vi "Open FP.vi"(8 "error in (no error)":errorcluster, 11 "AMS Gas Actor in":refnum<class "AMS Gas Actor.lvclass">=refnum) -> (0 "error out":errorcluster, 3 "AMS Gas Actor out":refnum<class "AMS Gas Actor.lvclass">)   [LabVIEW 2015]
uses:
  AMS Gas Actor.lvclass
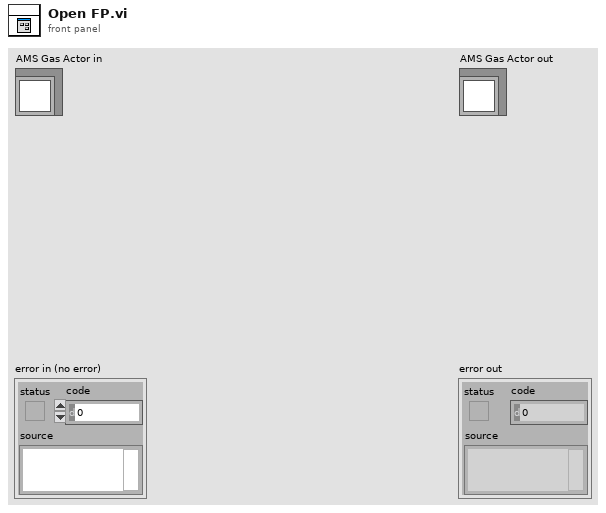
[diagram p1: front panel]
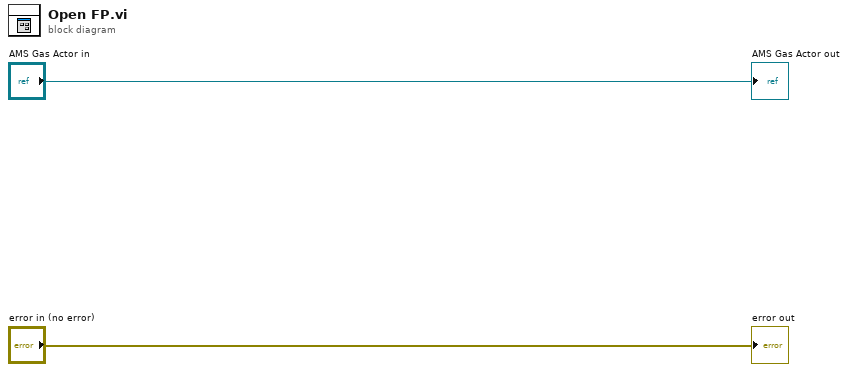
[diagram p0: block diagram]
diagram:
  "error out" <- "error in (no error)"
  "AMS Gas Actor out" <- "AMS Gas Actor in"
